vi "ReadWriteTest.vi"(8 "error in (no error)":errorcluster) -> (0 "error out":errorcluster)   [LabVIEW 2023, in "TestVIs.lvlib"]
uses:
  <vilib>/addons/_JKI Toolkits/Caraya/classes/Assert/Assert Equal Value_Variant.vi
  TestVIs.lvlib
  <vilib>/addons/_JKI Toolkits/Caraya/classes/Assert/Assert.lvclass
  <vilib>/addons/_JKI Toolkits/Caraya/classes/Test/Test.lvclass
  Library/Unit Testing CA1.lvlib
panel:
  # "READ WRITE TEST"
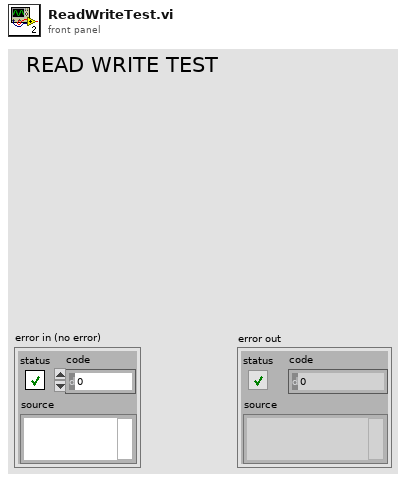
[diagram p1: front panel]
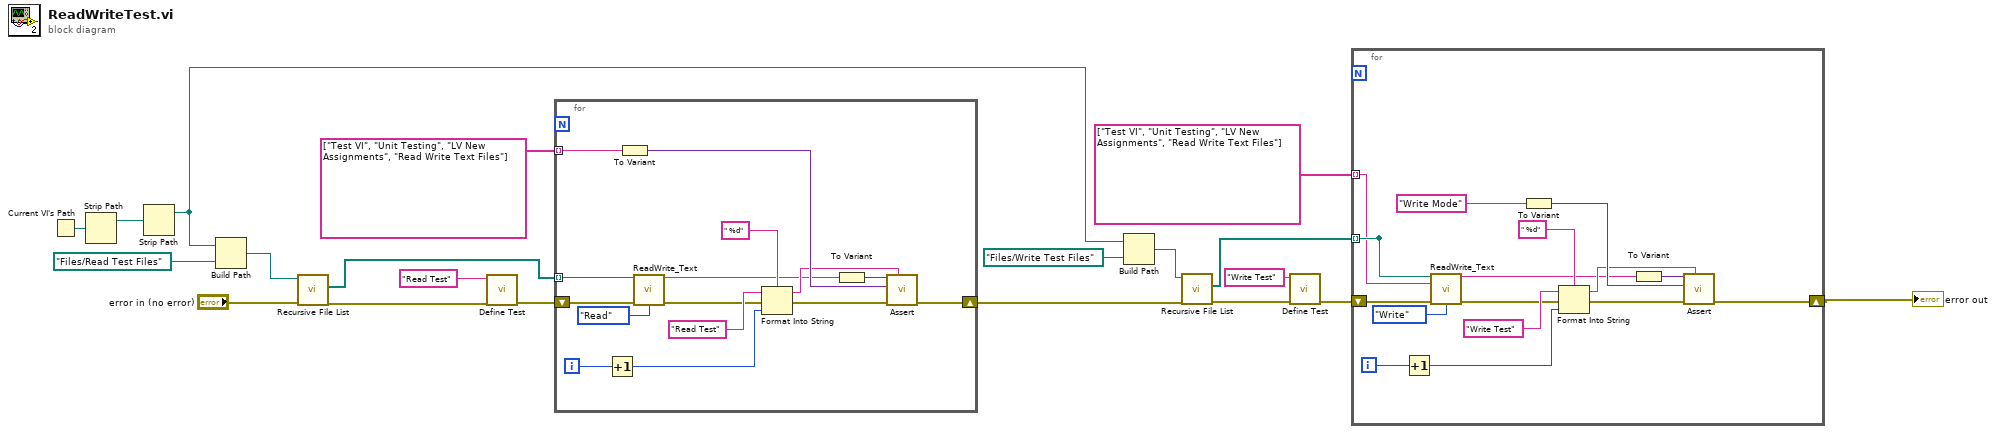
[diagram p0: block diagram]
diagram:
  n1 = Current VI's Path() -> (path=w20:path)
  n2 = Strip Path(path=w20) -> (stripped path=w16:path)  [unwired: 1 out]
  n3 = Strip Path(path=w16) -> (stripped path=w7:path)  [unwired: 1 out]
  n4 = Build Path(base path=w7, name or relative path=path "Files/Read Test Files") -> (appended path=w14:path)
  n5 = call <vilib>:"Recursive File List.vi"("error in (no error)"="error in (no error)", "Folder Path"=w14) -> ("error out"=w13:errorcluster, "All Files in Dir"=w11:path[])  [unwired: 5 in, 3 out]
  n6 = call <vilib>:"Define Test.vi"("error in (no error)"=w13, "Label (VI Title)"="Read Test") -> ("error out"=w17:errorcluster)  [unwired: 8 in, 1 out]
  n7 = for {
    tunnel: w11 -> [w25] mode=indexing
    shift-right: [w23] -> w6
    shift-left: w17 -> [w27]
    tunnel: string[] ["Test VI", "Unit Testing", "LV New Assignments", "Read Write Text Files"] ("Array") -> [w35] mode=indexing
    i -> [w30]
    n8 = Increment(x=w30) -> (x+1=w24:i32)
    n9 = To Variant(anything=w35) -> (Variant=w34:variant)
    n10 = call "ReadWrite_Text.vi"("file path"=w25, "error in"=w27, "Read/Write"=enum16{"Read", "Write"}."Read") -> ("Read String"=w22:string, "error out"=w26:errorcluster)  [unwired: 11 in]
    n11 = Format Into String(format string=" %d", initial string="Read Test" ("Label"), error in=w26, w24) -> (resulting string=w28:string, error out=w32:errorcluster)
    n12 = To Variant(anything=w22) -> (Variant=w33:variant)
    n13 = call-poly <vilib>:"Assert.vi"("Label"=w28, "error in (no error)"=w32, "Y"=w34, "X"=w33) -> ("error out"=w23:errorcluster)  [unwired: 6 in, 1 out]
  }
  n14 = Build Path(base path=w7, name or relative path=path "Files/Write Test Files") -> (appended path=w3:path)
  n15 = call <vilib>:"Recursive File List.vi"("error in (no error)"=w6, "Folder Path"=w3) -> ("error out"=w5:errorcluster, "All Files in Dir"=w4:path[])  [unwired: 5 in, 3 out]
  n16 = call <vilib>:"Define Test.vi"("error in (no error)"=w5, "Label (VI Title)"="Write Test") -> ("error out"=w9:errorcluster)  [unwired: 8 in, 1 out]
  n17 = for {
    tunnel: [w38] -> _ mode=indexing
    shift-right: [w41] -> w1
    shift-left: w9 -> [w44]
    tunnel: w4 -> [w38] mode=indexing
    tunnel: string[] ["Test VI", "Unit Testing", "LV New Assignments", "Read Write Text Files"] ("Array") -> [w37] mode=indexing
    i -> [w47]
    n18 = Increment(x=w47) -> (x+1=w42:i32)
    n19 = call "ReadWrite_Text.vi"("file path"=w38, "Write String"=w37, "error in"=w44, "Read/Write"=enum16{"Read", "Write"}."Write") -> ("Read String"=w40:string, "error out"=w43:errorcluster)  [unwired: 10 in]
    n20 = To Variant(anything="Write Mode" ("File/Folder Name")) -> (Variant=w51:variant)
    n21 = Format Into String(format string=" %d", initial string="Write Test" ("Label"), error in=w43, w42) -> (resulting string=w45:string, error out=w49:errorcluster)
    n22 = To Variant(anything=w40) -> (Variant=w50:variant)
    n23 = call-poly <vilib>:"Assert.vi"("Label"=w45, "error in (no error)"=w49, "Y"=w51, "X"=w50) -> ("error out"=w41:errorcluster)  [unwired: 6 in, 1 out]
  }
  "error out" <- w1
